vi "Failure Popup.vi"(11 "Logger in":refnum<class "Logger.lvclass">) -> ()   [LabVIEW 2018, in "Logging.lvlib" / "Logger.lvclass"]
uses:
  Logger.lvclass
  Logger.lvclass/Logger.ctl
  <vilib>/Utility/error.llb/DialogType.ctl
  <vilib>/addons/_JKI.lib/Serialization/JSON/Library/Timestamp Options.ctl
  <vilib>/addons/_JKI.lib/Serialization/JSON/JKI JSON Serialization.lvlib
  Utilities/Utilities.lvlib
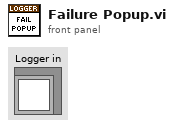
[diagram p1: front panel]
types:
  T1 = typedef "DialogType.ctl" = u16
  T2 = typedef "JKI JSON Serialization.lvlib/Timestamp Options.ctl" = cluster{"Convert Timestamps":bool, "UTC":bool}
  T3 = typedef "Logging.lvlib/Internal Log Levels.ctl" = enum16{"Trace", "Debug", "Info", "Warning", "Error", "Critical", "Internal"}
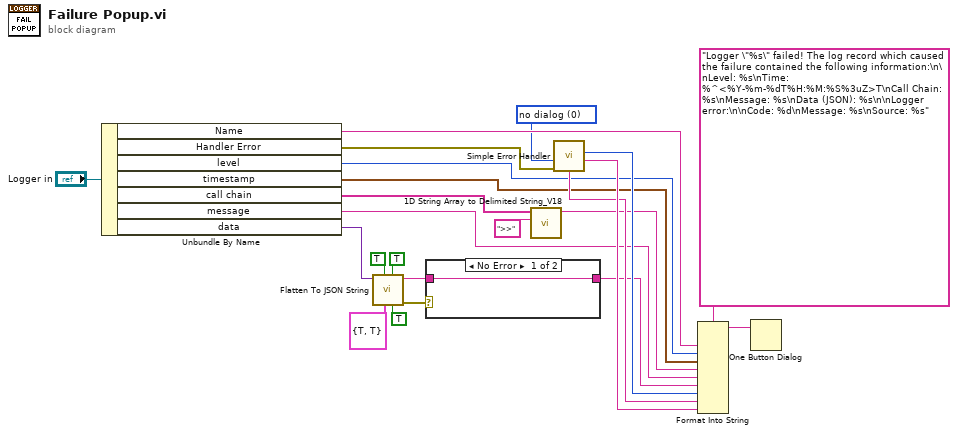
[diagram p0: block diagram]
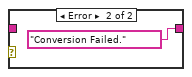
[diagram p2: hidden frame]
diagram:
  w13 = T1 0 items=["no dialog", "OK message", "continue or stop message", "OK message + warnings", "continue/stop + warnings"] ("type of dialog (OK msg:1)")
  n1 = Unbundle By Name("Logger in") -> ("Name"=w15:string, "Handler Error"=w7:errorcluster, "level"=w16:T3, "timestamp"=w17:timestamp, "call chain"=w8:string[], "message"=w19:string, "data"=w5:variant)
  n2 = call <vilib>:"Flatten To JSON String.vi"("Enums As String (F)"=TRUE, "Numeric Extensions (F)"=TRUE, "Timestamp Options"=T2 {"Convert Timestamps"=TRUE, "UTC"=TRUE}, "Multiline (T)"=TRUE, "Variant"=w5) -> ("error out"=w10:errorcluster, "JSON String"=w11:string)  [unwired: 5 in]
  n3 = case shown="No Error" w10 {
    tunnel: w11 -> [w24 _]
    tunnel: [w24 "Conversion Failed." ("JSON String")] -> w20
    frame No Error {
    }
    frame Error {
    }
  }
  n4 = call "1D String Array to Delimited String_V18.vi"("delimiter"=">>", "string array"=w8) -> ("delimited string"=w18:string)  [unwired: 9 in]
  n5 = call <vilib>:"Simple Error Handler.vi"("type of dialog (OK msg:1)"=w13, "error in (no error)"=w7) -> ("code out"=w21:i32, "source out"=w23:string, "message"=w22:string)  [unwired: 3 in, 2 out]
  n6 = Format Into String(format string="Logger \"%s\" failed! The log record which caused the failure contained the following information:\n\nLevel: %s\nTime: %^<%Y-%m-%dT%H:%M:%S%3uZ>T\nCall Chain: %s\nMessage: %s\nData (JSON): %s\n\nLogger error:\n\nCode: %d\nMessage: %s\nSource: %s", w15, w16, w17, w18, w19, w20, w21, w22, w23) -> (resulting string=w12:string)  [unwired: 2 in, 1 out]
  n7 = One Button Dialog(message=w12) -> ()  [unwired: 1 in, 1 out]
